vi "Obtain-settings-file-paths-with-dialog.vi"(8 "error in":errorcluster, 11 "Data ref. in":refnum<data-value>) -> (0 "error IO":errorcluster, 1 "Path ok?":bool, 2 "File paths":path[](array[path]), 3 "Data ref.":refnum<data-value>)   [LabVIEW 2013, in "CameraVision.lvlib" / "CV-Main.lvclass"]
doc: "This function determines whether the save is programmatically started (start of acquisition) or not, by checking the enabled state of the 'Start' button. Enabled means a user initiated save.\n\nIn case of an automated save the returned file paths are that of the user-selected storage directory with the base file name, appended with the file extension (.xml) and that of the directory and default name of the last-used-settings file (<Application>\\Program data\\last.xml).\n\nIn the case of a user save a dialog is displayed to ask the user to choose a filepath and name.\n\nWhen a file with the same path and name already exists, a warning message is displayed which allows the user to cancel or confirm the save operation."
uses:
  CV-Main.lvclass
  UI/Popup-messages.ctl
  UI/CV-UI.lvclass
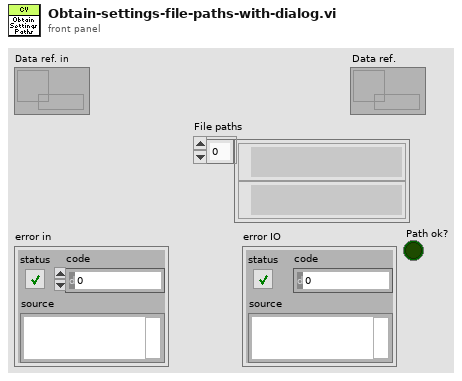
[diagram p1: front panel]
types:
  T1 = typedef "CameraVision.lvlib/CV-UI.lvclass/Popup-messages.ctl" = enum16{"Error-Black image", "Error-Camera config file", "Error-Camera connect", "Error-Grabber init", "Error-Camera setting", "Error-Image offset", "Error-Image import", "Error-Settings file not exist", "Error-Timing source", "Conflict-Filters", "Conflict-Map", "Conflict-Framerate", "Conflict-Charact", "Conflict-Temperature field", "Conflict-Temperature value", "Conflict-Storage-Binary image", "Conflict-Storage-Corrected image", "Conflict-Storage-Map", "Conflict-Storage-Charact", "Conflict-Storage-Temperature field", "Conflict-Storage-Temperature value", "Warning-File exist", "Warning-Parameter reset", "Warning-User cancel", "Info-Images imported"}
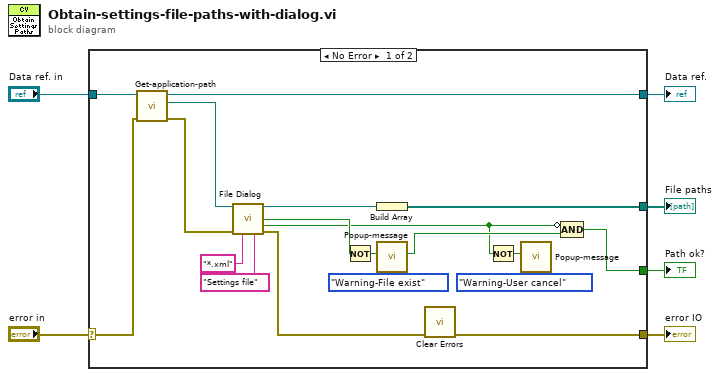
[diagram p0: block diagram]
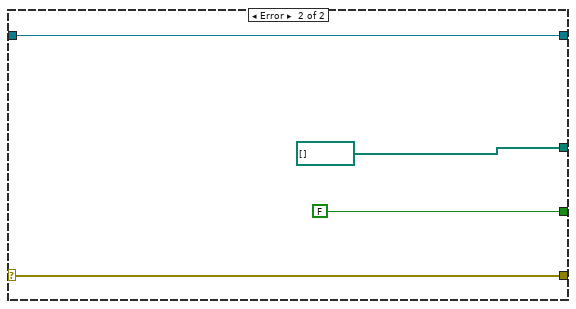
[diagram p2: hidden frame]
diagram:
  n1 = case shown="No Error" "error in" {
    selector: "error in" -> [w15 w29]
    tunnel: [w25 FALSE ("T button?")] -> w6
    tunnel: [w24 path[] []] -> w5
    tunnel: [w23 w29] -> w3
    tunnel: "Data ref. in" -> [w17 w27]
    tunnel: [w18 w27] -> w1
    frame No Error {
      n2 = call "Get-application-path.vi"("error in (no error)"=w15, "Data ref. in"=w17) -> ("error out"=w14:errorcluster, "App path"=w16:path, "Data ref."=w18:refnum<data-value>)  [unwired: 7 in]
      n3 = call "File Dialog"("start path"=w16, "error in"=w14, "pattern (all files)"="*.xml", "pattern label"="Settings file") -> ("selected path"=w21:path, "exists"=w20:bool, "cancelled"=w9:bool, "error out"=w13:errorcluster)  [unwired: 8 in]
      n4 = Not(x=w20) -> (.not. x?=w8:bool)
      n5 = Build Array(w21) -> (w24:path[])
      n6 = call "Popup-message.vi"("Message"=Popup-messages."Warning-File exist", "Ignore?"=w8) -> ("Return"=w10:bool)  [unwired: 9 in]
      n7 = call <vilib>:"Clear Errors.vi"("error in (no error)"=w13) -> ("error out"=w23:errorcluster)  [unwired: 6 in]
      n8 = Not(x=w9) -> (.not. x?=w7:bool)
      n9 = call "Popup-message.vi"("Message"=Popup-messages."Warning-User cancel", "Ignore?"=w7) -> ()  [unwired: 9 in, 1 out]
      n10 = Compound Arithmetic op=AND(invert w9, w10) -> (w25:bool)
    }
    frame Error {
    }
  }
  "Path ok?" <- w6
  "File paths" <- w5
  "error IO" <- w3
  "Data ref." <- w1
